vi "macro_LinearSystemLoop_DCMotor_Execute.vi"   [LabVIEW 2019, in "Trajectory_Library.lvlib"]
uses:
  Trajectory_Library.lvlib
  Enum/DCMOTOR_TYPES_ENUM.ctl
types:
  T1 = typedef "Trajectory_Library.lvlib/DCMOTOR_TYPES_ENUM.ctl" = enum16{"CIM", "AndyMark 9015", "Andy Mark RS 775 125", "Bag", "BaneBots RS 550", "BaneBots RS 775", "Falcon 500", "Mini CIM", "NEO", "NEO 550", "Romi BuiltIn", "Vex 775 Pro", "Snow Blower AM 2235A", "Bosch Seat AM 3493"}
  T2 = typedef "Trajectory_Library.lvlib/LINEAR_SYSTEM_ID_DCMOTOR_MODEL.ctl" = cluster{"DCMOTOR_TYPES":T1, "Num Motors":i32, "Gearing":dbl, "MOI kgm2":dbl}
  T3 = typedef "Trajectory_Library.lvlib/LINEAR_SYSTEM_LOOP_DCMOTOR_CTRL_PARAMS.ctl" = cluster{"Vel Model Std Dev Rad/Sec":dbl, "Vel Meas Std Dev Rad/Sec":dbl, "Vel Ctrl Tol Rad/Sec":dbl, "Max Ctrl Out V":dbl, "Pos Model Std Dev Rad":dbl, "Pos Meas Std Dev Rad":dbl, "Pos Ctrl Tol Rad":dbl}
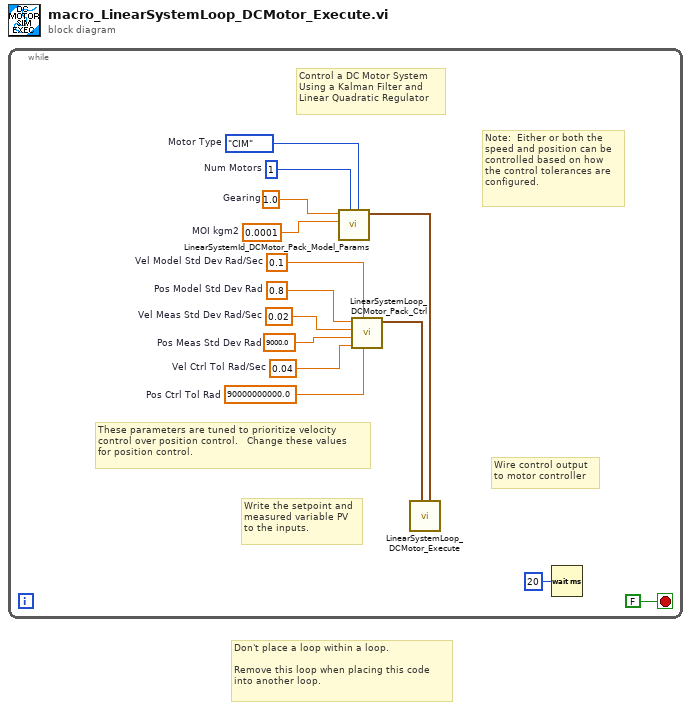
[diagram p0: block diagram]
diagram:
  # "Don't place a loop within a loop.\n \nRemove this loop when placing this code\ninto another loop."
  n1 = while {
    stop <- FALSE stop-if-true
    w1 = 0.8  # Pos Model Std Dev Rad
    w2 = 0.02  # Vel Meas Std Dev Rad/Sec
    w3 = 9000.0  # Pos Meas Std Dev Rad
    w4 = 0.04  # Vel Ctrl Tol Rad/Sec
    w5 = 0.1  # Vel Model Std Dev Rad/Sec
    w6 = 90000000000.0  # Pos Ctrl Tol Rad
    w11 = 1.0  # Gearing
    w12 = 0.0001  # MOI kgm2
    w13 = 1  # Num Motors
    w14 = DCMOTOR_TYPES_ENUM."CIM"  # Motor Type
    # "These parameters are tuned to prioritize velocity\ncontrol over position control.   Change these values\nfor position control."
    # "Write the setpoint and\nmeasured variable PV\nto the inputs."
    # "Wire control output\nto motor controller"
    # "Note:  Either or both the\nspeed and position can be\ncontrolled based on how\nthe control tolerances are\nconfigured."
    # "Control a DC Motor System\nUsing a Kalman Filter and \nLinear Quadratic Regulator"
    n2 = call "LinearSystemId_DCMotor_Pack_Model_Params.vi"("DCMOTOR_TYPES"=w14, "Num Motors"=w13, "MOI kgm2"=w12, "Gearing"=w11) -> ("LinearSystem_ID_DCMotor_Model"=w8:T2)  [unwired: 7 in]
    n3 = call "LinearSystemLoop_DCMotor_Pack_Ctrl.vi"("Pos Ctrl Tol Rad"=w6, "Vel Model Std Dev Rad/Sec"=w5, "Vel Ctrl Tol Rad/Sec"=w4, "Pos Meas Std Dev Rad"=w3, "Vel Meas Std Dev Rad/Sec"=w2, "Pos Model Std Dev Rad"=w1) -> ("LinearSystemLoop_DCMotor_Ctrl_Params"=w7:T3)  [unwired: 5 in]
    n4 = call "LinearSystemLoop_DCMotor_Execute.vi"("LinearSystem_ID_DCMotor_Model"=w8, "LinearSystem_DCMotor_Ctrl_Params"=w7) -> ()  [unwired: 5 in, 5 out]
    n5 = Wait (ms)(milliseconds to wait=u32 20) -> ()  [unwired: 1 out]
  }
